vi "admin.vi"(11 "Password":string) -> ()   [LabVIEW 2021]
uses:
  controls/Control 1.ctl
panel:
  in  "?":string
  in  "?":string
  in  "?":string
  in  "?":string
  in  "?":string
  in  "?":string
  in  "?":string
  in  "?":string
  in  "Min":string
  in  "?":string
  in  "?":string
  in  "?":string
  in  "?":string
  in  "?":string
  in  "?":string
  in  "?":string
  in  "?":string
  in  "Temp sensor":T1
  in  "Update":bool
  out "error out":errorcluster
  out "appended array":string[](array[string])
  in  "Max":string
  in  "Min":string
  in  "Max":string
  in  "Min":string
  in  "Max":string
  in  "Min 1":string
  in  "Max":string
  in  "Min":string
  in  "Max":string
  in  "Min":string
  in  "Max":string
  in  "error in":errorcluster
  # "Insulation Resistance"
  # "Weld Resistance Test"
  # "Cell 1 - End Busbar"
  # "Temperature Harness Test-Imbalance"
  # "Cell 1 - Cell 2"
  # "Cell 2 - Cell 3"
  # "Cell Voltage"
  # "Cell 3 - Cell 4"
  # "Cell 4 - Cell 5"
  # "Voltage Harness Test"
  # "Cell 5 - Cell 6"
  # "Temperature Harness Test-Ambient"
  # "Cell 6 - Cell 7"
  # "Cell 7 - Cell 8"
  # "Temperature Sensor"
  # "Cell 8 - End Busbar"
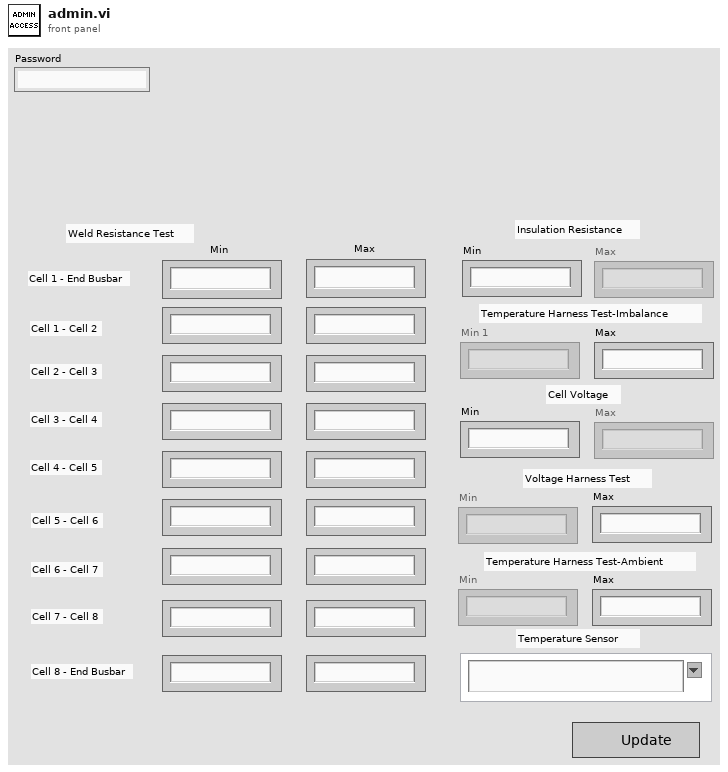
[diagram p1: front panel]
types:
  T1 = typedef "Control 1.ctl" = string
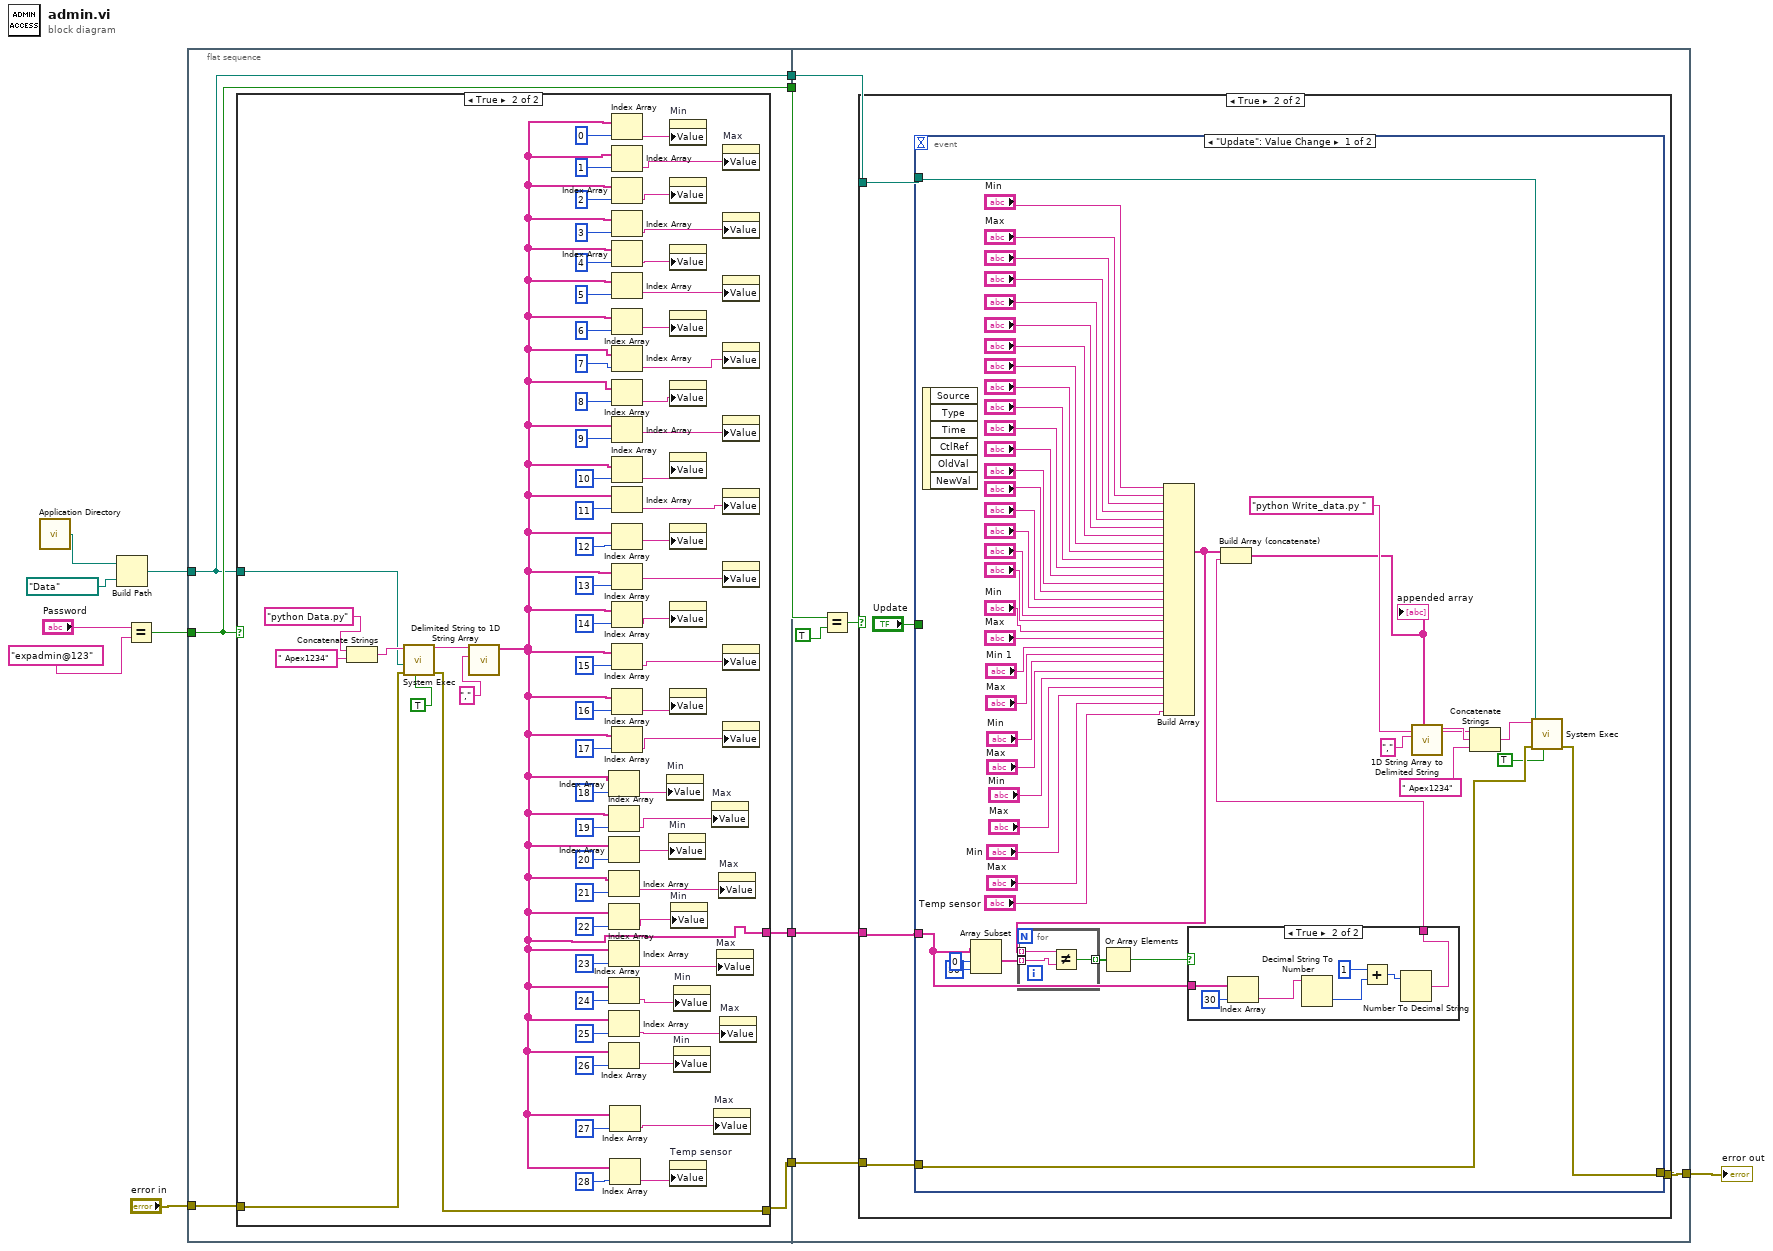
[diagram p0: block diagram]
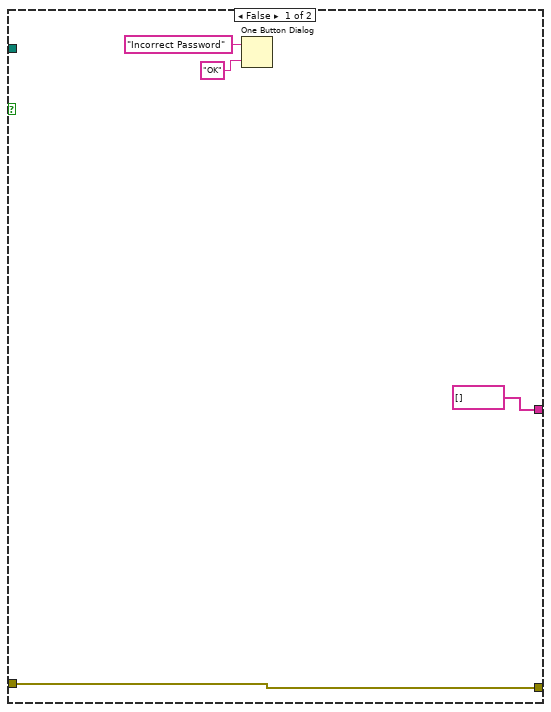
[diagram p2: hidden frame]
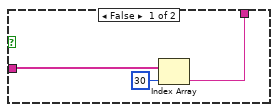
[diagram p4: hidden frame]
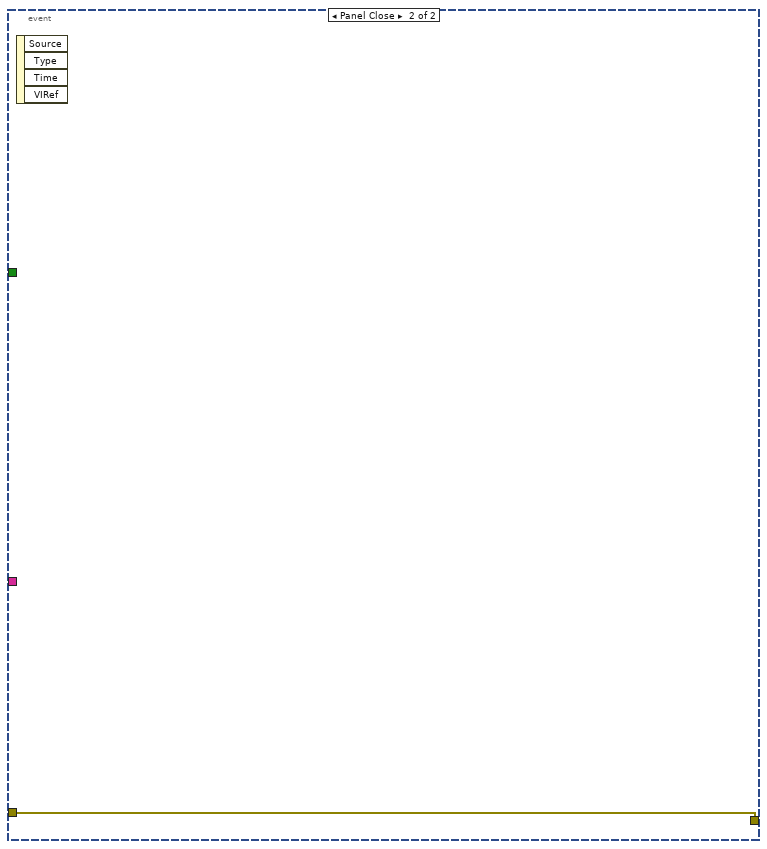
[diagram p5: hidden frame]
diagram:
  n1 = call <vilib>:"Application Directory.vi"() -> ("Application Directory"=w2:path)
  n2 = Build Path(base path=w2, name or relative path=path "Data" ("working directory")) -> (appended path=w1:path)
  n3 = Equal?(x="Password", y="expadmin@123") -> (x = y?=w10:bool)
  n4 = flat-sequence {
    tunnel: [w17] -> w12
    tunnel: w10 -> [w16]
    tunnel: [w16] -> w9
    tunnel: w1 -> [w14]
    tunnel: [w14] -> w5
    tunnel: [w15] -> w4
    tunnel: "error in" -> [w13]
    tunnel: w12 -> [w96]
    tunnel: [w95] -> w8
    tunnel: w9 -> [w90]
    tunnel: w5 -> [w92]
    tunnel: w4 -> [w91]
    frame #0 {
      n5 = case shown="True" w16 {
        tunnel: w13 -> [w21 w89]
        tunnel: [w21 w88] -> w17
        tunnel: w14 -> [_ w68]
        tunnel: [string[] [] ("string array") w30] -> w15
        frame False {
          n6 = One Button Dialog(message="Incorrect Password", button name ("OK")="OK") -> ()  [unwired: 1 out]
        }
        frame True {
          n7 = Concatenate Strings("python Data.py" ("command line"), " Apex1234" ("string")) -> (w70:string)
          n8 = call <vilib>:"System Exec.vi"("run minimized? (F)"=TRUE, "error in (no error)"=w89, "working directory"=w68, "command line"=w70) -> ("error out"=w88:errorcluster, "standard output"=w87:string)  [unwired: 4 in, 2 out]
          n9 = call <vilib>:"Delimited String to 1D String Array.vi"("delimiter"=",", "delimited string"=w87) -> ("string array"=w30:string[])  [unwired: 9 in]
          n10 = Index Array(array=w30, index=18) -> (element=w64:string)
          n11 = Index Array(array=w30, index=19) -> (element=w63:string)
          n12 = Index Array(array=w30, index=20) -> (element=w29:string)
          n13 = Index Array(array=w30, index=21) -> (element=w28:string)
          n14 = Index Array(array=w30, index=22) -> (element=w27:string)
          n15 = Index Array(array=w30, index=23) -> (element=w26:string)
          n16 = Index Array(array=w30, index=24) -> (element=w25:string)
          n17 = Index Array(array=w30, index=25) -> (element=w24:string)
          n18 = Index Array(array=w30, index=26) -> (element=w23:string)
          n19 = Index Array(array=w30, index=27) -> (element=w22:string)
          n20 = Index Array(array=w30, index=28) -> (element=w65:string)
          n21 = Index Array(array=w30, index=0) -> (element=w48:string)
          n22 = Index Array(array=w30, index=1) -> (element=w47:string)
          n23 = Index Array(array=w30, index=2) -> (element=w46:string)
          n24 = Index Array(array=w30, index=3) -> (element=w45:string)
          n25 = Index Array(array=w30, index=4) -> (element=w44:string)
          n26 = Index Array(array=w30, index=5) -> (element=w43:string)
          n27 = Index Array(array=w30, index=6) -> (element=w42:string)
          n28 = Index Array(array=w30, index=7) -> (element=w41:string)
          n29 = Index Array(array=w30, index=8) -> (element=w40:string)
          n30 = Index Array(array=w30, index=9) -> (element=w39:string)
          n31 = Index Array(array=w30, index=10) -> (element=w38:string)
          n32 = Index Array(array=w30, index=11) -> (element=w37:string)
          n33 = Index Array(array=w30, index=12) -> (element=w36:string)
          n34 = Index Array(array=w30, index=13) -> (element=w35:string)
          n35 = Index Array(array=w30, index=14) -> (element=w34:string)
          n36 = Index Array(array=w30, index=15) -> (element=w33:string)
          n37 = Index Array(array=w30, index=16) -> (element=w32:string)
          n38 = Index Array(array=w30, index=17) -> (element=w31:string)
          n39 = property on="Min" class="Str"("Value"=w64) -> ()  [unwired: 2 in, 2 out]
          n40 = property on="Min" class="Str"("Value"=w29) -> ()  [unwired: 2 in, 2 out]
          n41 = property on="Min" class="Str"("Value"=w48) -> ()  [unwired: 2 in, 2 out]
          n42 = property class="Str"("Value"=w46) -> ()  [unwired: 2 in, 2 out]
          n43 = property class="Str"("Value"=w44) -> ()  [unwired: 2 in, 2 out]
          n44 = property class="Str"("Value"=w42) -> ()  [unwired: 2 in, 2 out]
          n45 = property class="Str"("Value"=w40) -> ()  [unwired: 2 in, 2 out]
          n46 = property class="Str"("Value"=w38) -> ()  [unwired: 2 in, 2 out]
          n47 = property class="Str"("Value"=w36) -> ()  [unwired: 2 in, 2 out]
          n48 = property class="Str"("Value"=w34) -> ()  [unwired: 2 in, 2 out]
          n49 = property class="Str"("Value"=w32) -> ()  [unwired: 2 in, 2 out]
          n50 = property on="Temp sensor" class="CmbBox (strict)"("Value"=w65) -> ()  [unwired: 2 in, 2 out]
          n51 = property on="Min" class="Str"("Value"=w27) -> ()  [unwired: 2 in, 2 out]
          n52 = property on="Min" class="Str"("Value"=w25) -> ()  [unwired: 2 in, 2 out]
          n53 = property on="Min" class="Str"("Value"=w23) -> ()  [unwired: 2 in, 2 out]
          n54 = property on="Max" class="Str"("Value"=w63) -> ()  [unwired: 2 in, 2 out]
          n55 = property on="Max" class="Str"("Value"=w22) -> ()  [unwired: 2 in, 2 out]
          n56 = property on="Max" class="Str"("Value"=w26) -> ()  [unwired: 2 in, 2 out]
          n57 = property on="Max" class="Str"("Value"=w28) -> ()  [unwired: 2 in, 2 out]
          n58 = property on="Max" class="Str"("Value"=w24) -> ()  [unwired: 2 in, 2 out]
          n59 = property on="Max" class="Str"("Value"=w47) -> ()  [unwired: 2 in, 2 out]
          n60 = property class="Str"("Value"=w45) -> ()  [unwired: 2 in, 2 out]
          n61 = property class="Str"("Value"=w43) -> ()  [unwired: 2 in, 2 out]
          n62 = property class="Str"("Value"=w41) -> ()  [unwired: 2 in, 2 out]
          n63 = property class="Str"("Value"=w39) -> ()  [unwired: 2 in, 2 out]
          n64 = property class="Str"("Value"=w37) -> ()  [unwired: 2 in, 2 out]
          n65 = property class="Str"("Value"=w35) -> ()  [unwired: 2 in, 2 out]
          n66 = property class="Str"("Value"=w33) -> ()  [unwired: 2 in, 2 out]
          n67 = property class="Str"("Value"=w31) -> ()  [unwired: 2 in, 2 out]
        }
      }
    }
    frame #1 {
      n68 = Equal?(x=w90, y=TRUE) -> (x = y?=w93:bool)
      n69 = case shown="True" w93 {
        tunnel: [w97 w101] -> w95
        tunnel: w96 -> [w97 w102]
        tunnel: w92 -> [_ w98]
        tunnel: w91 -> [_ w99]
        frame False {
        }
        frame True {
          n70 = event shown="[0] \"Update\": Value Change" {
            selector: _ -> [_ _]
            dyn-events: _ -> [_ _]
            timeout: _ -> [_ _]
            tunnel: w102 -> [w149 w163]
            tunnel: [w148 w163] -> w101
            tunnel: "Update" -> [_ _]
            tunnel: w98 -> [w142 _]
            tunnel: w99 -> [w105 _]
            event "Update": Value Change {
              n71 = event-data() -> ()  [unwired: 1 in, 6 out]
              n72 = Array Subset(array=w105, index=0, length=30) -> (w106:string[])
              n73 = Build Array("Min", "Max", "?", "?", "?", "?", "?", "?", "?", "?", "?", "?", "?", "?", "?", "?", "?", "?", "Min", "Max", "Min 1", "Max", "Min", "Max", "Min", "Max", "Min", "Max", "Temp sensor") -> (w108:T1[])
              n74 = for {
                tunnel: [w152] -> w138 mode=indexing
                tunnel: w108 -> [w151] mode=indexing
                tunnel: w106 -> [w150] mode=indexing
                n75 = Not Equal?(x=w151, y=w150) -> (x != y?=w152:bool)
              }
              n76 = Or Array Elements(Boolean array=w138) -> (logical OR=w107:bool)
              n77 = case shown="True" w107 {
                tunnel: w105 -> [w155 w161]
                tunnel: [w153 w156] -> w140
                frame False {
                  n78 = Index Array(array=w155, index=30) -> (element=w153:string)
                }
                frame True {
                  n79 = Index Array(array=w161, index=30) -> (element=w160:string)
                  n80 = Decimal String To Number(string=w160) -> (number=w159:i32)  [unwired: 2 in, 1 out]
                  n81 = Add(x=1, y=w159) -> (x+y=w157:i32)
                  n82 = Number To Decimal String(number=w157) -> (decimal integer string=w156:string)  [unwired: 1 in]
                }
              }
              n83 = Build Array (concatenate)(w108, w140) -> (w139:T1[])
              "appended array" <- w139
              n84 = call <vilib>:"1D String Array to Delimited String.vi"("delimiter"=",", "string array"=w139) -> ("delimited string"=w147:string)  [unwired: 9 in]
              n85 = Concatenate Strings("python Write_data.py " ("command line"), w147, " Apex1234" ("string")) -> (w144:string)
              n86 = call <vilib>:"System Exec.vi"("run minimized? (F)"=TRUE, "error in (no error)"=w149, "working directory"=w142, "command line"=w144) -> ("error out"=w148:errorcluster)  [unwired: 4 in, 3 out]
            }
            event Panel Close {
              n87 = event-data() -> ()  [unwired: 1 in, 4 out]
            }
          }
        }
      }
    }
  }
  "error out" <- w8
